vi "pi_piezo_to_xml.vi"(8 "error in":errorcluster, 11 "PI Piezo Settings":T1) -> (0 "error out":errorcluster, 3 "PI piezo settings string":string)   [LabVIEW 2012]
uses:
  settings.ctl
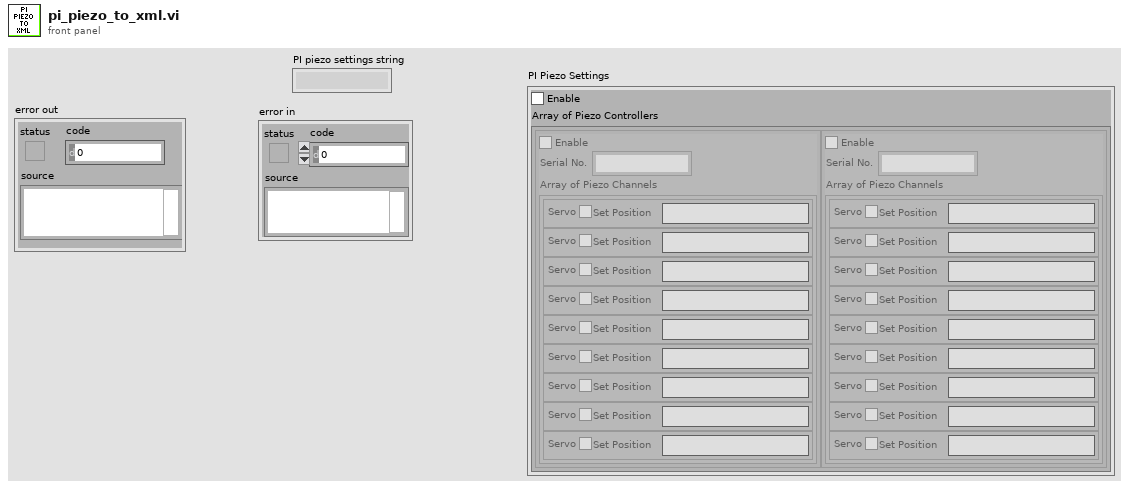
[diagram p1: front panel]
types:
  T1 = typedef "settings.ctl" = cluster{"Enable":bool, "Array of Piezo Controllers":cluster{"Enable":bool, "Serial No.":string, "Array of Piezo Channels":cluster{"Servo":bool, "Set Position":string}[]}[]}
  T2 = cluster{"Enable":bool, "Serial No.":string, "Array of Piezo Channels":cluster{"Servo":bool, "Set Position":string}[]}[]
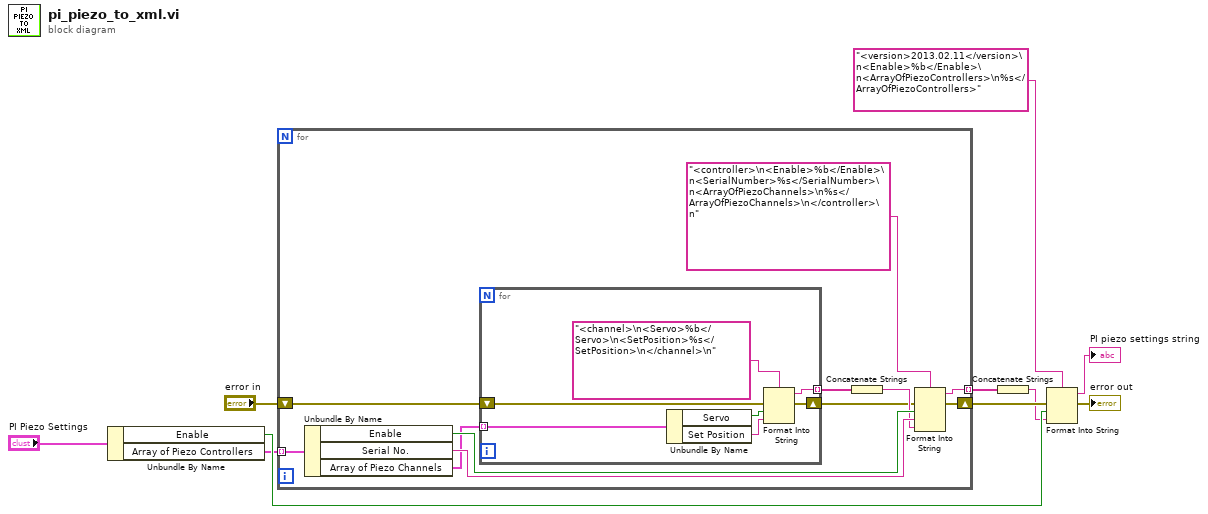
[diagram p0: block diagram]
diagram:
  n1 = Unbundle By Name("PI Piezo Settings") -> ("Enable"=w9:bool, "Array of Piezo Controllers"=w7:T2)
  n2 = for {
    tunnel: w7 -> [w21] mode=indexing
    shift-right: [w17] -> w5
    shift-left: "error in" -> [w12]
    tunnel: [w16] -> w4 mode=indexing
    n3 = Unbundle By Name(w21) -> ("Enable"=w20:bool, "Serial No."=w19:string, "Array of Piezo Channels"=w15:cluster{"Servo":bool, "Set Position":string}[])
    n4 = for {
      tunnel: w15 -> [w24] mode=indexing
      tunnel: [w27] -> w14 mode=indexing
      shift-right: [w25] -> w11
      shift-left: w12 -> [w26]
      n5 = Unbundle By Name(w24) -> ("Servo"=w23:bool, "Set Position"=w22:string)
      n6 = Format Into String(format string="<channel>\n<Servo>%b</Servo>\n<SetPosition>%s</SetPosition>\n</channel>\n", error in=w26, w23, w22) -> (resulting string=w27:string, error out=w25:errorcluster)  [unwired: 1 in]
    }
    n7 = Concatenate Strings(w14) -> (w13:string)
    n8 = Format Into String(format string="<controller>\n<Enable>%b</Enable>\n<SerialNumber>%s</SerialNumber>\n<ArrayOfPiezoChannels>\n%s</ArrayOfPiezoChannels>\n</controller>\n", error in=w11, w20, w19, w13) -> (resulting string=w16:string, error out=w17:errorcluster)  [unwired: 1 in]
  }
  n9 = Concatenate Strings(w4) -> (w3:string)
  n10 = Format Into String(format string="<version>2013.02.11</version>\n<Enable>%b</Enable>\n<ArrayOfPiezoControllers>\n%s</ArrayOfPiezoControllers>", error in=w5, w9, w3) -> (resulting string=→"PI piezo settings string":string, error out=→"error out":errorcluster)  [unwired: 1 in]
